vi "InitAction.vi"(6 "InstrumentName":string, 7 "VisaRessIn":refnum<visa-resource-name>, 8 "error in (no error)":errorcluster caption="entrée d'erreur (pas d'erreur)", 9 "FirstClassInst":bool, 10 "Function":string, 11 "GenData In":refnum<class "Triax320.lvclass"> caption="DNL_LabVIEW Object in") -> (0 "error out":errorcluster caption="sortie d'erreur", 3 "GenData Out":refnum<class "Triax320.lvclass"> caption="DNL_LabVIEW Object out")   [LabVIEW 2019, in "Triax320.lvclass"]
uses:
  Triax320.lvclass
  C:/Programmes LabView/LabScanV1A/DevicesClass/BaseDevice/BaseDevice.lvclass
  Triax320_Func.ctl
  Triax320.lvclass/Triax320.ctl
panel:
  in  "DefaultDev_Func":T1
  out "VisaRessOut":refnum<visa-resource-name>
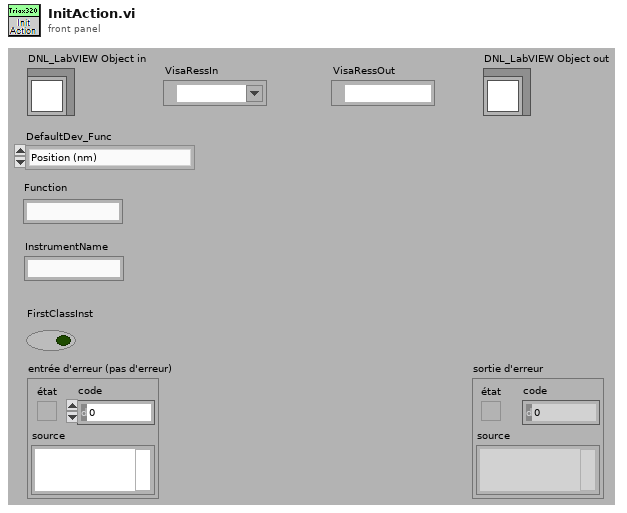
[diagram p1: front panel]
types:
  T1 = typedef "Triax320.lvclass/Triax320_Func.ctl" = enum16{"Position (nm)"}
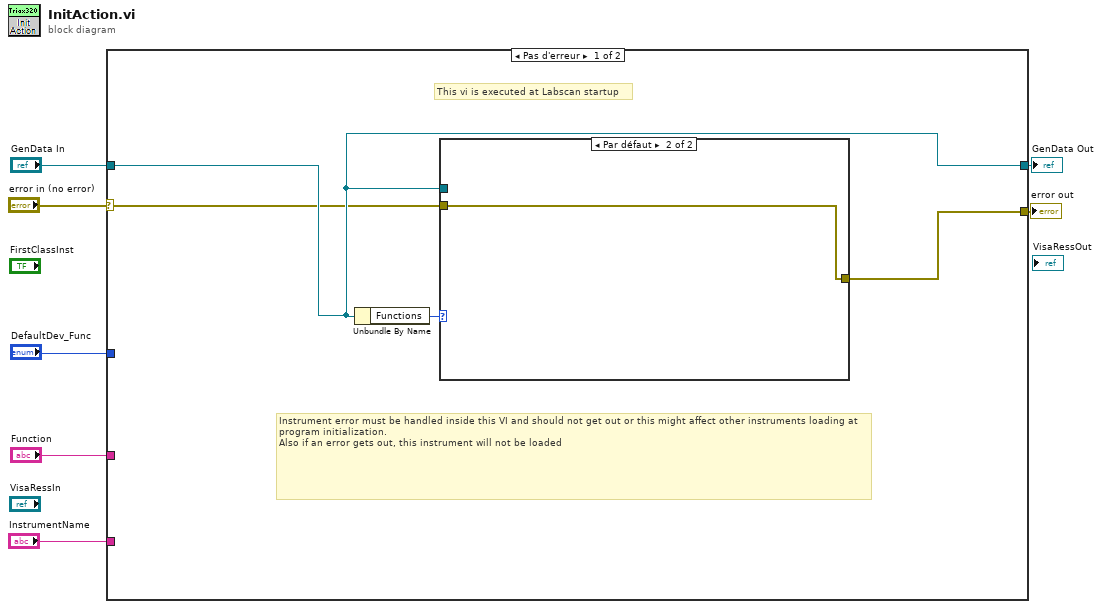
[diagram p0: block diagram]
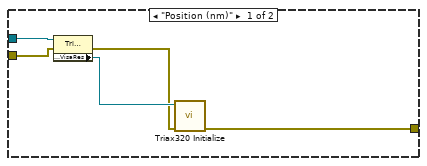
[diagram p2: hidden frame]
diagram:
  n1 = case shown="Pas d'erreur" "error in (no error)" {
    selector: "error in (no error)" -> [w9 w19]
    tunnel: [w8 w19] -> w6
    tunnel: "GenData In" -> [w10 w18]
    tunnel: [w10 w18] -> w4
    tunnel: "DefaultDev_Func" -> [_ _]
    tunnel: "Function" -> [_ _]
    tunnel: "InstrumentName" -> [_ _]
    frame No Error {
      # "This vi is executed at Labscan startup"
      # "Instrument error must be handled inside this VI and should not get out or this might affect other instruments loading at program initialization.\nAlso if an error gets out, this instrument will not be loaded"
      n2 = Unbundle By Name(w10) -> ("Functions"=w11:T1)
      n3 = case shown="Par défaut" w11 {
        tunnel: w10 -> [w16 _]
        tunnel: w9 -> [w15 w17]
        tunnel: [w12 w17] -> w8
        frame "Position (nm)" {
          n4 = property class="Triax320.lvclass"(reference=w16, error in=w15) -> (error out=w13:errorcluster, "Accessor:VisaRes"=w14:refnum<visa-resource-name>)  [unwired: 1 out]
          n5 = call <userlib>:"Triax320 Initialize.vi"("error in (no error)"=w13, "Triax VISA Rsrc"=w14) -> ("error out"=w12:errorcluster)  [unwired: 7 in, 2 out]
        }
        frame Default {
        }
      }
    }
    frame Error {
    }
  }
  "error out" <- w6
  "GenData Out" <- w4
